vi "Read Justify tabs.vi"(9 "Tab in":refnum<class "Tab.lvclass">) -> (3 "Tab out":refnum<class "Tab.lvclass">, 4 "Justify tabs":bool)   [LabVIEW 2014, in "Tab.lvclass"]
uses:
  Tab.lvclass
  Tab.lvclass/Tab.ctl
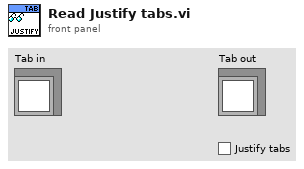
[diagram p1: front panel]
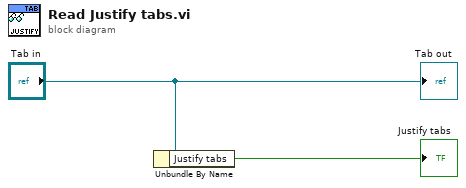
[diagram p0: block diagram]
diagram:
  n1 = Unbundle By Name("Tab in") -> ("Justify tabs"=→"Justify tabs":bool)
  "Tab out" <- "Tab in"
